vi "First Step.vi"(8 "error in (no error)":errorcluster, 11 "Wavelength.lvclass in":refnum<class "Wavelength Triax 550.lvclass">) -> (0 "error out":errorcluster, 2 "Current Position":dbl, 3 "Wavelength.lvclass out":refnum<class "Wavelength Triax 550.lvclass">)   [LabVIEW 2017, in "Wavelength Triax 550.lvclass"]
uses:
  Wavelength Triax 550.lvclass
  Instruments/Spectrometer Triax 550/Spectrometer Triax 550.lvclass
  C:/LabVIEW-programs/Instruments/Utility Classes/Scannable/Scannable.lvclass
  Scanner/Scanner.lvclass
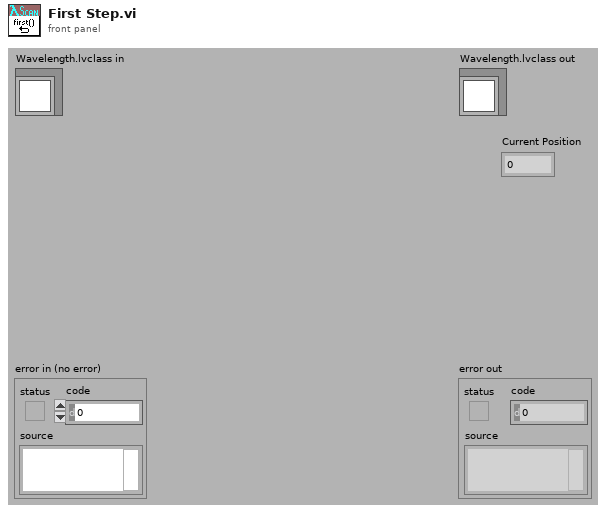
[diagram p1: front panel]
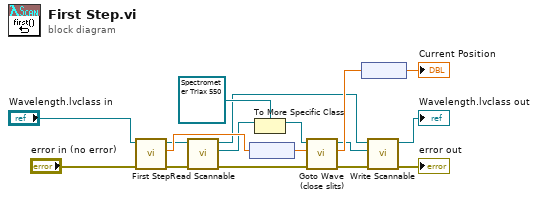
[diagram p0: block diagram]
diagram:
  n1 = call-parent "First Step.vi"("error in (no error)"="error in (no error)", "Scanner.lvclass in"="Wavelength.lvclass in") -> ("error out"=w11:errorcluster, "Current Position"=w15:dbl, "Scanner.lvclass out"=w9:refnum<class "Wavelength Triax 550.lvclass">)  [unwired: 7 out]
  n2 = call-dynamic "Read Scannable.vi"("error in (no error)"=w11, "Scanner.lvclass in"=w9) -> ("error out"=w10:errorcluster, "Scannable.lvclass"=w6:refnum<class "Scannable.lvclass">, "Scanner.lvclass out"=w2:refnum<class "Wavelength Triax 550.lvclass">)  [unwired: 7 out]
  n3 = node(w15) -> (w12:dbl[unit])
  n4 = To More Specific Class(target class=refnum<class "Spectrometer Triax 550.lvclass"> refnum ("Spectrometer Triax 550.lvclass"), reference=w6) -> (specific class reference=w5:refnum<class "Spectrometer Triax 550.lvclass">)  [unwired: 1 in, 1 out]
  n5 = call "Goto Wave (close slits).vi"("error in (no error)"=w10, "Target Wavelength"=w12, "Spectrometer Triax 550 in"=w5) -> ("error out"=w1:errorcluster, "Actual Wavelength"=w13:dbl[unit], "Spectrometer Triax 550 out"=w3:refnum<class "Spectrometer Triax 550.lvclass">)  [unwired: 6 out]
  n6 = node(w13) -> (→"Current Position":dbl)
  n7 = call-dynamic "Write Scannable.vi"("error in (no error)"=w1, "Scannable.lvclass"=w3, "Scanner.lvclass in"=w2) -> ("error out"=→"error out":errorcluster, "Scanner.lvclass out"=→"Wavelength.lvclass out":refnum<class "Wavelength Triax 550.lvclass">)  [unwired: 7 out]
